vi "WaitForStartup.vi"(3 "ROS":T1={"topic port"=0, "Node"="", "topic"="", "type"="", "node port"=0, "error "={"status"=FALSE, "code"=0, "source"=""}, "Direction"=enum."Node", "Update (ms)"=1, "FIFO size"=1}) -> (1 "success?":bool)   [LabVIEW 2018]
doc: "Waits for a new topic"
uses:
  <userlib>/ROS for LabVIEW Software/ROS/Code/SubVIs/_ROSControl.ctl
  <userlib>/ROS for LabVIEW Software/ROS/Code/SubVIs/_ROSDirection.ctl
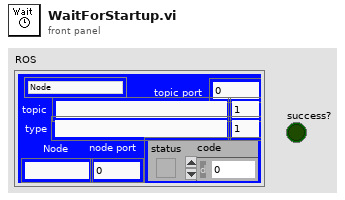
[diagram p1: front panel]
types:
  T1 = typedef "_ROSControl.ctl" = cluster{"topic port":u16, "Node":string, "topic":string, "type":string, "node port":u16, "error ":errorcluster, "Direction":T2, "Update (ms)":u16, "FIFO size":u16}
  T2 = typedef "_ROSDirection.ctl" = enum16{"Node", "Publisher", "Subscriber", "ServiceClient", "ServiceProvider"}
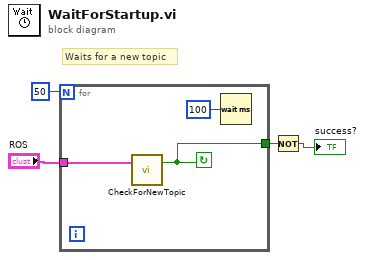
[diagram p0: block diagram]
diagram:
  # "Waits for a new topic"
  n1 = for {
    N: 50 -> [_]
    tunnel: "ROS" -> [w6]
    tunnel: [w5] -> w1
    stop <- w5 continue-if-true
    n2 = call <userlib>:"CheckForNewTopic.vi"("ROS"=w6) -> ("new?"=w5:bool)  [unwired: 2 in]
    n3 = Wait (ms)(milliseconds to wait=u32 100) -> ()  [unwired: 1 out]
  }
  n4 = Not(x=w1) -> (.not. x?=→"success?":bool)
